vi "Hamamatsu_Init.vi"(0 "object in":refnum<class "Hamamatsu.lvclass">, 2 "Image Type":T1=7 items=["Grayscale (U8)", "Grayscale (I16)", "Grayscale (SGL)", "Complex (CSG)", "RGB (U32)", "HSL (U32)", "RGB (U64)", "Grayscale (U16)"], 5 "error in (no error)":errorcluster) -> (14 "object out":refnum<class "Hamamatsu.lvclass">, 19 "error out":errorcluster)   [LabVIEW 2021, in "Hamamatsu.lvclass"]
uses:
  Hamamatsu.lvclass
  Hamamatsu.lvclass/Hamamatsu.ctl
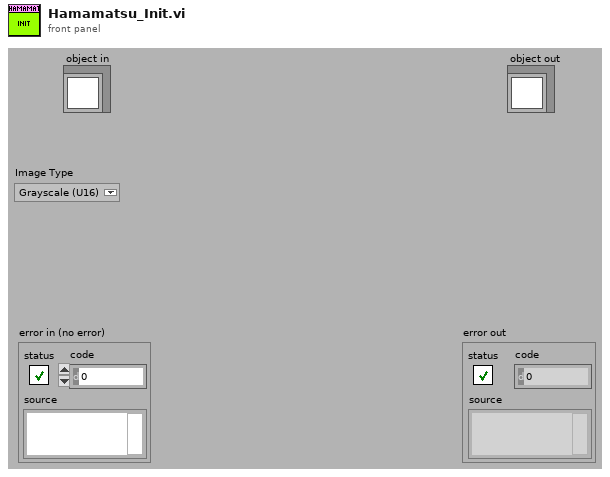
[diagram p1: front panel]
types:
  T1 = typedef "Image Type" = u32
  T2 = cluster{"Capture Library":string, "DCAM-API":string}
  T3 = typedef "IMAQ Image.ctl" = refnum<image>
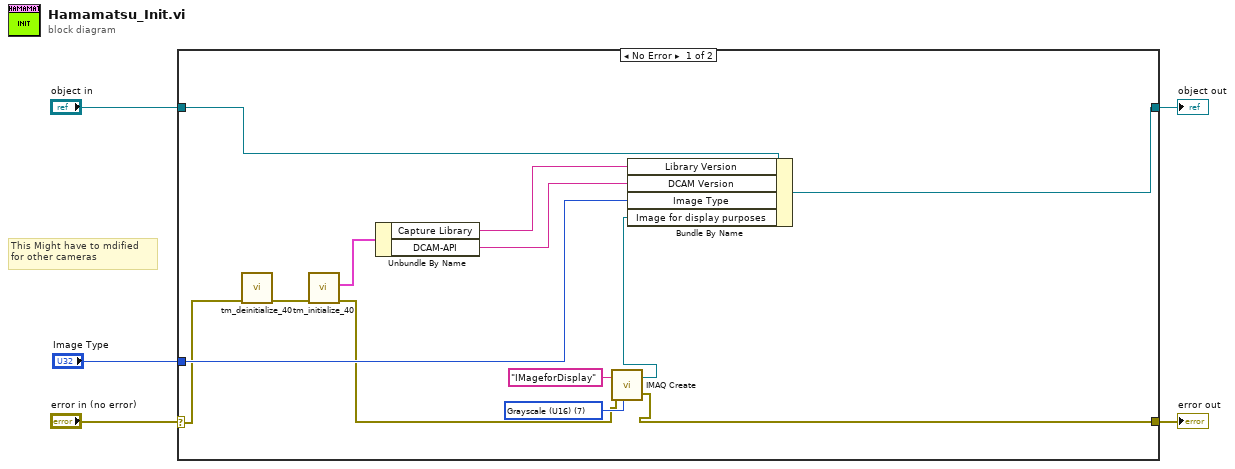
[diagram p0: block diagram]
diagram:
  # "This Might have to mdified \nfor other cameras"
  n1 = case shown="No Error" "error in (no error)" {
    selector: "error in (no error)" -> [w12 w19]
    tunnel: [w18 w20] -> w5
    tunnel: "object in" -> [w17 w20]
    tunnel: [w6 w19] -> w2
    tunnel: "Image Type" -> [w13 _]
    frame No Error {
      w8 = T1 7 items=["Grayscale (U8)", "Grayscale (I16)", "Grayscale (SGL)", "Complex (CSG)", "RGB (U32)", "HSL (U32)", "RGB (U64)", "Grayscale (U16)"] ("Image Type")
      n2 = call <userlib>:"tm_deinitialize_40.vi"("error in (no error)"=w12) -> ("error out"=w11:errorcluster)  [unwired: 10 in]
      n3 = call <userlib>:"tm_initialize_40.vi"("error in (no error)"=w11) -> ("error out"=w7:errorcluster, "Version Info"=w16:T2)  [unwired: 7 in, 2 out]
      n4 = Unbundle By Name(w16) -> ("Capture Library"=w15:string, "DCAM-API"=w14:string)
      n5 = call "IMAQ Create"("Image Name"="IMageforDisplay", "Image Type"=w8, "error in (no error)"=w7) -> ("New Image"=w9:T3, "error out"=w6:errorcluster)  [unwired: 2 in]
      n6 = Bundle By Name(cluster=w17, "Library Version"=w15, "DCAM Version"=w14, "Image Type"=w13, "Image for display purposes"=w9) -> (w18:refnum<class "Hamamatsu.lvclass">)
    }
    frame Error {
    }
  }
  "object out" <- w5
  "error out" <- w2
